vi "Read Key (I32).vi"(7 "section":string, 8 "error in (no error)":errorcluster, 9 "default value":i32, 10 "key":string, 11 "refnum":T1) -> (0 "error out":errorcluster, 1 "value":i32, 2 "found?":bool, 3 "refnum out":T1)   [LabVIEW 2017, in "NI_LVConfig.lvlib"]
doc: "Reads a value associated with a key in a specified section from the configuration data identified by <B>refnum</B>. If the key does not exist, the VI returns the default value. This VI supports multibyte characters in strings. Wire data to the <B>default value</B> input to determine the polymorphic instance to use or manually select the instance."
uses:
  <vilib>/Utility/config.llb/NI_LVConfig.lvlib
  <vilib>/Utility/config.llb/Config Data RefNum.ctl
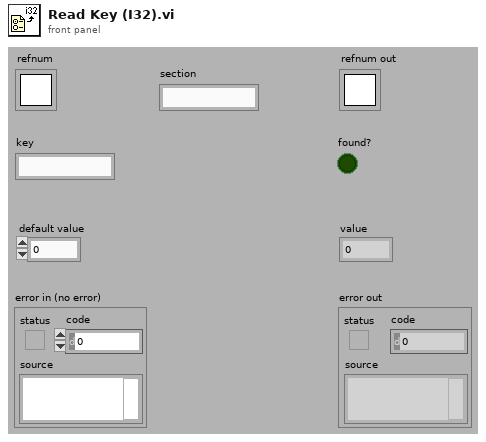
[diagram p1: front panel]
types:
  T1 = typedef "NI_LVConfig.lvlib/Config Data RefNum.ctl" = refnum<k1>
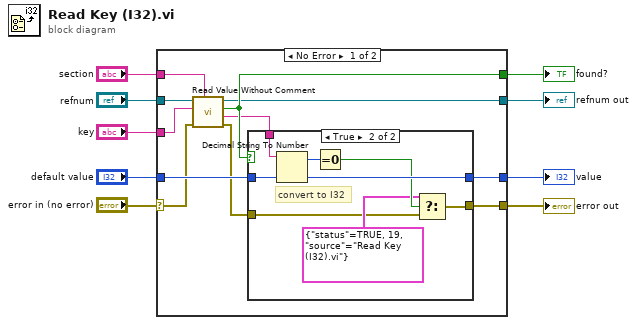
[diagram p0: block diagram]
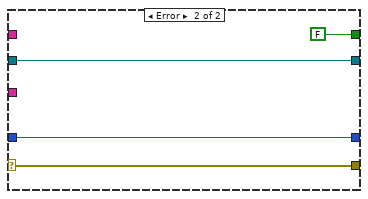
[diagram p3: hidden frame]
diagram:
  n1 = case shown="No Error" "error in (no error)" {
    selector: "error in (no error)" -> [w12 w34]
    tunnel: [w19 w34] -> w8
    tunnel: [w10 w31] -> w2
    tunnel: "section" -> [w13 _]
    tunnel: "key" -> [w14 _]
    tunnel: "default value" -> [w20 w33]
    tunnel: [w17 FALSE ("key exists?")] -> w4
    tunnel: [w18 w33] -> w3
    tunnel: "refnum" -> [w11 w31]
    frame No Error {
      n2 = call <vilib>:"Read Value Without Comment.vi"("section"=w13, "error in (no error)"=w12, "key"=w14, "refnum"=w11) -> ("error out"=w15:errorcluster, "value"=w16:string, "found?"=w17:bool, "refnum out"=w10:T1)  [unwired: 4 out]
      n3 = case shown="True" w17 {
        tunnel: [w22 w30] -> w18
        tunnel: w16 -> [_ w29]
        tunnel: w20 -> [w22 w28]
        tunnel: w15 -> [w21 w23]
        tunnel: [w21 w24] -> w19
        frame False {
        }
        frame True {
          # "convert to I32"
          n4 = Decimal String To Number(string=w29, default (0L)=w28) -> (offset past number=w27:i32, number=w30:i32)  [unwired: 1 out]
          n5 = Equal To 0?(x=w27) -> (x = 0?=w26:bool)
          n6 = Select(t=cluster{"status":bool, u16, "source":string} {"status"=TRUE, 19, "source"="Read Key (I32).vi"} ("f"), s=w26, f=w23) -> (s? t:f=w24:errorcluster)
        }
      }
    }
    frame Error {
    }
  }
  "error out" <- w8
  "value" <- w3
  "found?" <- w4
  "refnum out" <- w2
